vi "Assert Result.vi"(8 "error in (no error)":errorcluster, 9 "Mock":refnum<class "Mock.lvclass">, 10 "Status":T1(ring), 11 "LUnit Test Case In":refnum<class "Test Case.lvclass">) -> (0 "error out":errorcluster, 3 "LUnit Test Case Out":refnum<class "Test Case.lvclass">)   [LabVIEW 2020, in "Expectation Test.lvclass"]
uses:
  Expectation Test.lvclass
  source/Framework/Mock/Mock.lvclass
  <vilib>/Astemes/LUnit/Test Case.lvclass
  <vilib>/Astemes/LUnit/Test Case.lvclass/Test Case.ctl
  c46993f4-e485-4ac3-9b25-20f97047735b.vi
  <vilib>/Astemes/LUnit/Append Pass Result.vi
  <vilib>/Astemes/LUnit/Append Fail Result.vi
  <vilib>/Astemes/LUnit/Describe Comparison.vi
  <vilib>/Astemes/LUnit/Compare Variants.vi
  <vilib>/Astemes/LUnit/Variant to string.vi
  <vilib>/Utility/Data Type/Get Type Information.vi
  <vilib>/Utility/LVClass/Get LV Class Name.vi
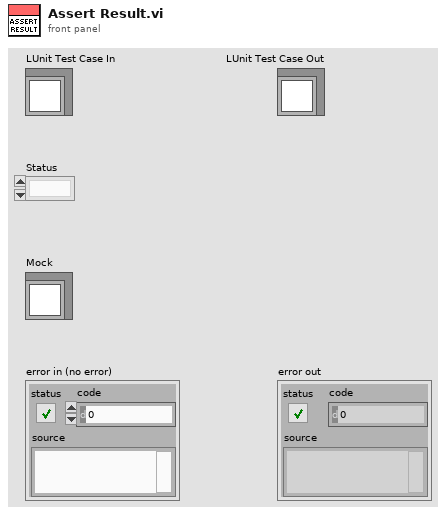
[diagram p1: front panel]
types:
  T1 = enum16{"", "Passed", "Failed", "Error", "Skipped", "Setup Error", "Broken", "Teardown Error"}
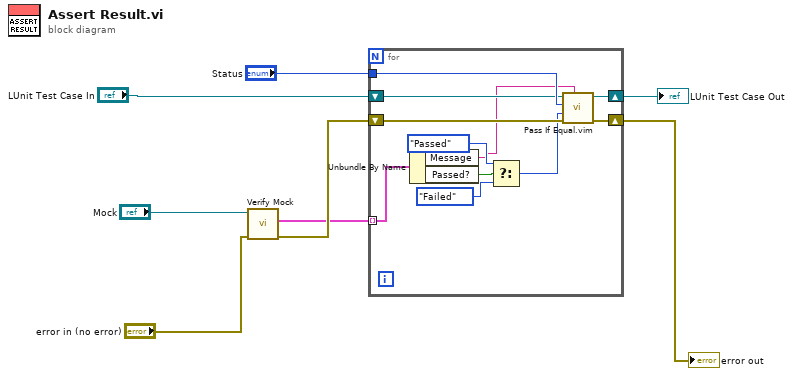
[diagram p0: block diagram]
diagram:
  n1 = call-dynamic "Verify Mock.vi"("error in (no error)"="error in (no error)", "Mock In"="Mock") -> ("error out"=w4:errorcluster, "Results"=w1:cluster{"Passed?":bool, "Message":string}[])  [unwired: 7 in, 1 out]
  n2 = for {
    tunnel: "Status" -> [w19]
    shift-right: [w18] -> w7
    shift-left: w4 -> [w17]
    shift-right: [w15] -> w2
    shift-left: "LUnit Test Case In" -> [w16]
    tunnel: w1 -> [w14] mode=indexing
    n3 = Unbundle By Name(w14) -> ("Message"=w9:string, "Passed?"=w13:bool)
    n4 = Select(t=T1."Passed" ("Status"), s=w13, f=T1."Failed" ("Status")) -> (s? t:f=w10:T1)
    n5 = call "Pass If Equal.vim"("Description"=w9, "error in (no error)"=w17, "Actual"=w10, "Expected"=w19, "LUnit Test Case In"=w16) -> ("error out"=w18:errorcluster, "LUnit Test Case Out"=w15:refnum<class "Test Case.lvclass">)  [unwired: 5 in]
  }
  "error out" <- w7
  "LUnit Test Case Out" <- w2
